vi "Error Converter (ErrCode or Status).vi"(8 "error in (no error)":errorcluster, 10 "Language":T1 items=["System dependent", "Not available", "Not available", "Not available", "Not available", "Not available", "Not available", "Deutsch", "Not available", "English", "Español", "Not available", "Français", "Not available", "Not available", "Not available", "Italiano"], 11 "error code":i32) -> (0 "error out":errorcluster)   [LabVIEW 2016]
uses:
  <instrlib>/KDI Digital Instrumentation/API_for_PCAN_BASIC_FD/Error language selector.ctl
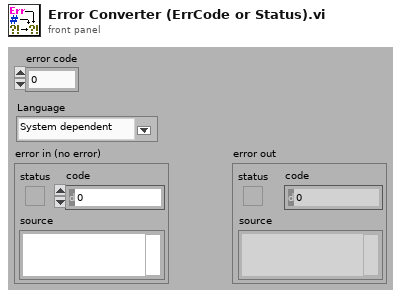
[diagram p1: front panel]
types:
  T1 = typedef "Error language selector.ctl" = u16
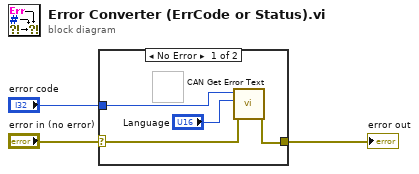
[diagram p0: block diagram]
diagram:
  n1 = case shown="No Error" "error in (no error)" {
    selector: "error in (no error)" -> [w5 w8]
    tunnel: [w4 w8] -> w2
    tunnel: "error code" -> [w7 _]
    frame No Error {
      n2 = call <instrlib>:"CAN Get Error Text.vi"("error in (no error)"=w5, "Language"="Language", "Error"=w7) -> ("error out"=w4:errorcluster)  [unwired: 8 in]
    }
    frame Error {
    }
  }
  "error out" <- w2
